vi "报警信息记录.vi"(6 "platform_alarm_code":string, 7 "参数":string, 8 "error in (no error)":errorcluster, 9 "code":u64, 10 "报警信息":string, 11 "Slave ID":T2=enum."氨氮") -> (0 "error out":errorcluster)   [LabVIEW 2016, in "质控单元V4.lvlib"]
panel:
  in  "data":T1={"时间"=timestamp(0 s since 1904-01-01), "参数"="水样测试", "报警信息"="N", "备注"="", "code"=0, "platform_alarm_code"=""}
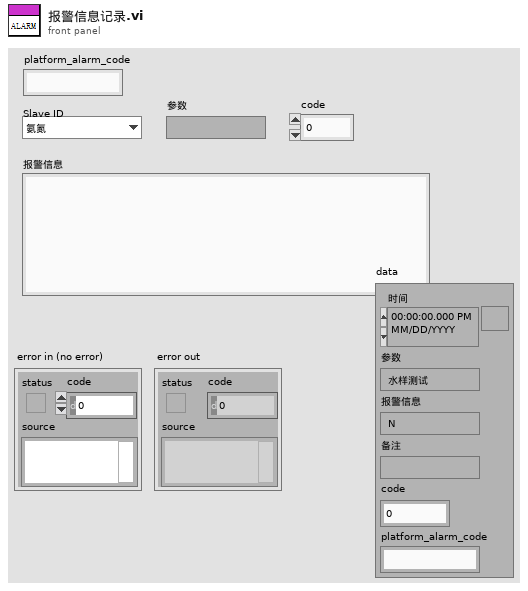
[diagram p1: front panel]
types:
  T1 = typedef "报警信息字段定义.ctl" = cluster{"时间":timestamp, "参数":string, "报警信息":string, "备注":string, "code":u64, "platform_alarm_code":string}
  T2 = typedef "质控单元V4.lvlib/质控slave id.ctl" = enum16{"null", "氨氮", "总磷", "总氮", "CODMn", "CODCr", "氟化物"}
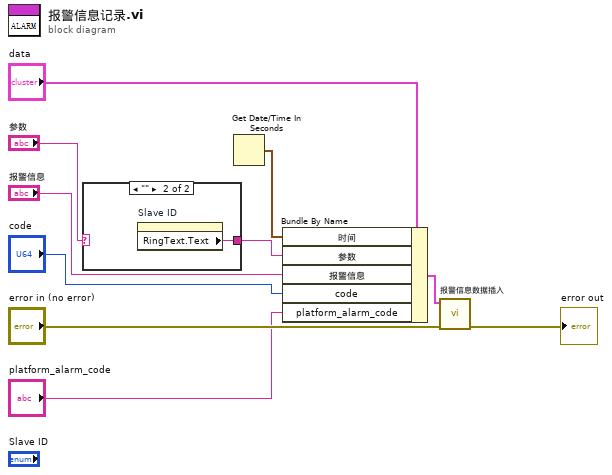
[diagram p0: block diagram]
diagram:
  n1 = case shown="\"\"" "参数" {
    selector: "参数" -> [w11 _]
    tunnel: [w11 w12] -> w4
    frame Default {
    }
    frame "" {
      n2 = property on="Slave ID" class="Enum (严格)"() -> ("RingText.Text"=w12:string)  [unwired: 2 in, 2 out]
    }
  }
  n3 = Get Date/Time In Seconds() -> (seconds since 1Jan1904=w10:timestamp)
  n4 = Bundle By Name(cluster="data", "时间"=w10, "参数"=w4, "报警信息"="报警信息", "code"="code", "platform_alarm_code"="platform_alarm_code") -> (w7:T1)
  n5 = call "报警信息数据插入.vi"("data"=w7, "错误输入（无错误）"="error in (no error)") -> ("错误输出"=→"error out":errorcluster)  [unwired: 8 in]
